vi "Generate selector strings.vi"(9 "[POI#] or [MiniScan#]":T1 {"ROI number" min=1 format="ROI %.0f"}, 10 "POI Averaged":bool, 11 "format string":string) -> (1 "[Visibility]":bool[](array[boolean]), 3 "Strings[]":string[](array[string]))   [LabVIEW 2013]
uses:
  Typedefs/ROI selector array-ROI vis.ctl
  xcontrol/Interface VIs/Interface typedefs/Interface-ROI selection cluster.ctl
  Typedefs/ROI ID Enum.ctl
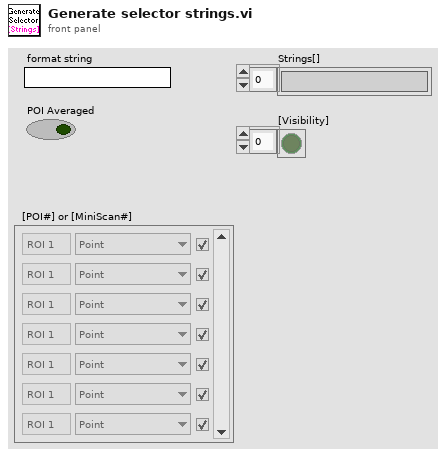
[diagram p1: front panel]
types:
  T1 = typedef "ROI selector array-ROI vis.ctl" = T2[]
  T2 = typedef "Interface-ROI selection cluster.ctl" = cluster{"ROI number":i32, "ROI ID":T3, "Visibility":bool}
  T3 = typedef "ROI ID Enum.ctl" = enum16{"Point", "MiniScan", "Comp. MiniScan", "Rectangle", "Comp. volume", "Arb. plane point"}
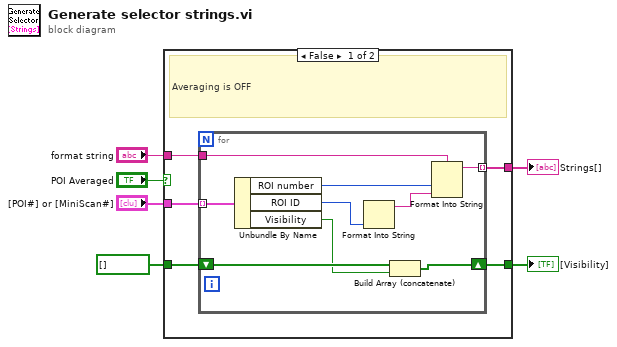
[diagram p0: block diagram]
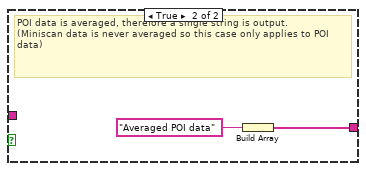
[diagram p2: hidden frame]
diagram:
  n1 = case shown="False" "POI Averaged" {
    tunnel: [w11 _] -> w6
    tunnel: bool[] [] -> [w10 _]
    tunnel: "[POI#] or [MiniScan#]" -> [w9 _]
    tunnel: "format string" -> [w8 _]
    tunnel: [w7 w21] -> w2
    frame False {
      # "Averaging is OFF"
      n2 = for {
        tunnel: w9 -> [w18] mode=indexing
        tunnel: [w19] -> w7 mode=indexing
        tunnel: w8 -> [w20]
        shift-right: [w17] -> w11
        shift-left: w10 -> [w16]
        n3 = Unbundle By Name(w18) -> ("ROI number"=w15:i32, "ROI ID"=w13:T3, "Visibility"=w14:bool)
        n4 = Format Into String(w13) -> (resulting string=w12:string)  [unwired: 3 in, 1 out]
        n5 = Build Array (concatenate)(w16, w14) -> (w17:bool[])
        n6 = Format Into String(format string=w20, w15, w12) -> (resulting string=w19:string)  [unwired: 2 in, 1 out]
      }
    }
    frame True {
      # "POI data is averaged, therefore a single string is output.\n(Miniscan data is never averaged so this case only applies to POI data)"
      n7 = Build Array("Averaged POI data") -> (w21:string[])
    }
  }
  "[Visibility]" <- w6
  "Strings[]" <- w2
